vi "LDA_U16_data_header.vi"() -> (0 "Output string":string)   [LabVIEW 2018]
uses:
  Globals/Meas_global.vi
  Globals/LDA_meas_global_1.vi
  Globals/LDA_meas_global_2.vi
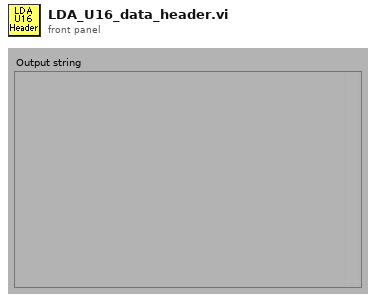
[diagram p1: front panel]
types:
  T1 = typedef "LDA_Setup.ctl" = cluster{"dimensions":enum16{"1D", "2D"}, "Sampling Rate Hz":dbl}
  T2 = typedef "BSA_Type.ctl" = enum16{"57N11", "BSA F60"}
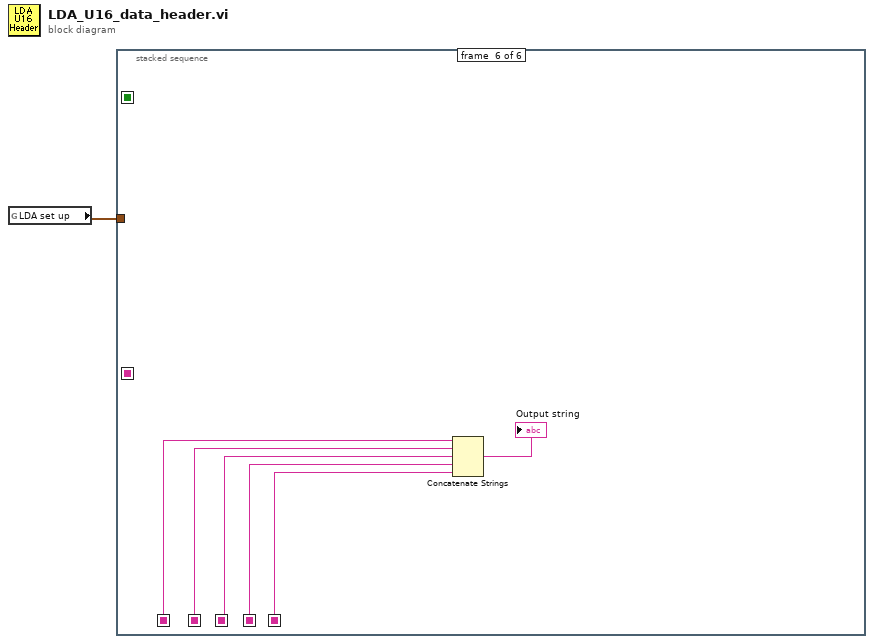
[diagram p0: block diagram]
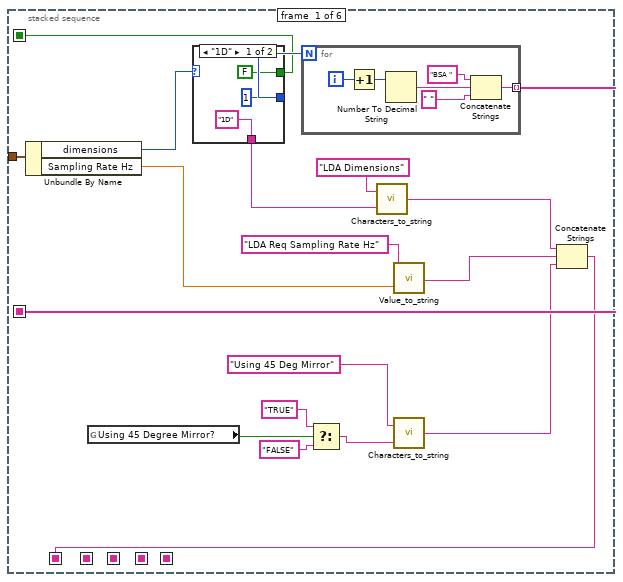
[diagram p2: hidden frame]
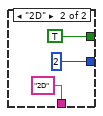
[diagram p3: hidden frame]
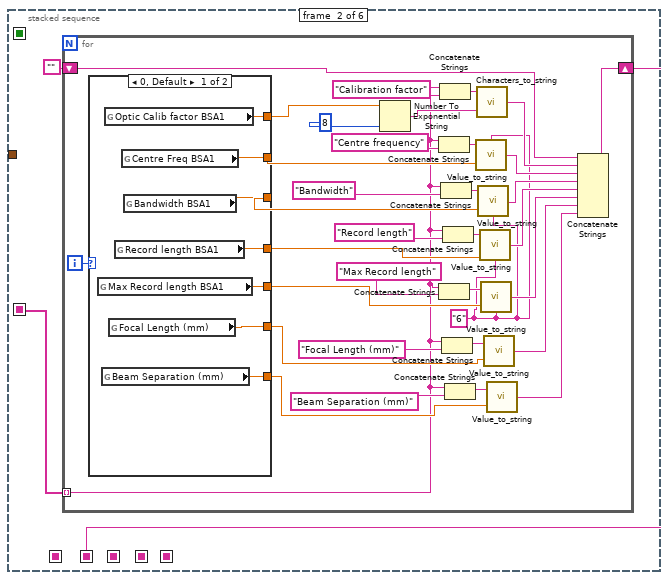
[diagram p4: hidden frame]
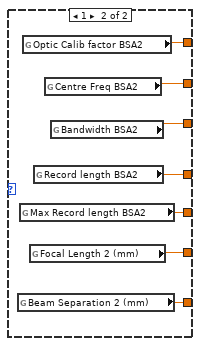
[diagram p5: hidden frame]
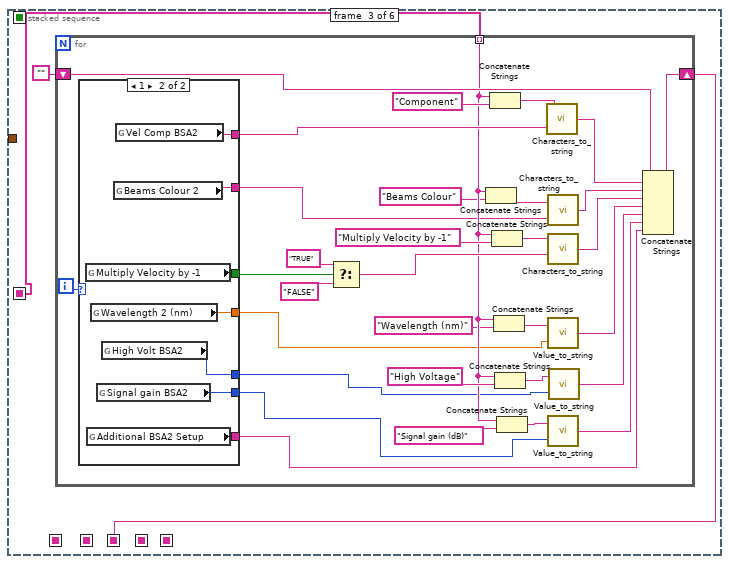
[diagram p6: hidden frame]
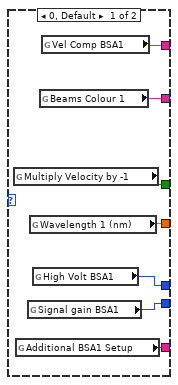
[diagram p7: hidden frame]
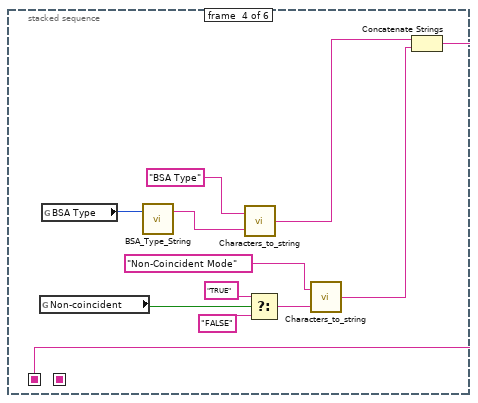
[diagram p8: hidden frame]
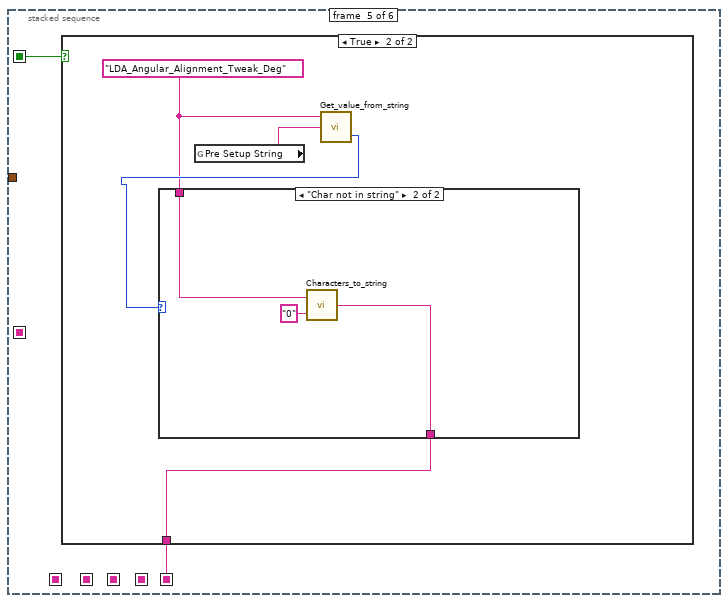
[diagram p9: hidden frame]
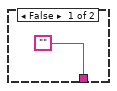
[diagram p10: hidden frame]
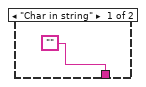
[diagram p11: hidden frame]
diagram:
  n1 = global read "Meas_global.vi" "LDA set up"() -> (w1:T1)
  n2 = stacked-sequence {
    seq-local: [_ w33 _ _ _ _] -> [_ _ _ _ _ w160]
    seq-local: [_ _ w85 _ _ _] -> [_ _ _ _ _ w159]
    seq-local: [w19 _ _ _ _ _] -> [_ w32 w84 _ _ _]
    seq-local: [_ _ _ w143 _ _] -> [_ _ _ _ _ w157]
    seq-local: [w2 _ _ _ _ _] -> [_ _ _ _ _ w156]
    seq-local: [_ _ _ _ w144 _] -> [_ _ _ _ _ w155]
    seq-local: [w11 _ _ _ _ _] -> [_ _ _ _ w145 _]
    tunnel: w1 -> [w10 _ _ _ _ _]
    frame #0 {
      n3 = Unbundle By Name(w10) -> ("dimensions"=w17:enum16{"1D", "2D"}, "Sampling Rate Hz"=w6:dbl)
      n4 = global read "LDA_meas_global_1.vi" "Using 45 Degree Mirror?"() -> (w13:bool)
      n5 = case shown="\"1D\"" w17 {
        tunnel: [1 2] -> w18
        tunnel: [FALSE TRUE] -> w11
        tunnel: ["1D" "2D"] -> w8
        frame "1D" {
        }
        frame "2D" {
        }
      }
      n6 = for {
        N: w18 -> [_]
        tunnel: [w28] -> w19 mode=indexing
        i -> [w26]
        n7 = Increment(x=w26) -> (x+1=w29:i32)
        n8 = Number To Decimal String(number=w29) -> (decimal integer string=w31:string)  [unwired: 1 out]
        n9 = Concatenate Strings("BSA ", w31, " ") -> (w28:string)
      }
      n10 = Select(t="TRUE", s=w13, f="FALSE") -> (s? t:f=w14:string)
      n11 = call "Characters_to_string.vi"("Characters to write"=w8, "Label for characters"="LDA Dimensions") -> ("Output string"=w5:string)
      n12 = call "Value_to_string.vi"("Value"=w6, "Label for value"="LDA Req Sampling Rate Hz") -> ("Output string"=w4:string)  [unwired: 1 in]
      n13 = call "Characters_to_string.vi"("Characters to write"=w14, "Label for characters"="Using 45 Deg Mirror") -> ("Output string"=w3:string)
      n14 = Concatenate Strings(w5, w4, w3) -> (w2:string)
    }
    frame #1 {
      n15 = for {
        shift-right: [w67] -> w33
        shift-left: "" -> [w68]
        tunnel: w32 -> [w35] mode=indexing
        i -> [w69]
        w47 = "6" ("precision")
        n16 = case shown="0, Default" w69 {
          tunnel: [w76 w80] -> w45
          tunnel: [w75 w81] -> w60
          tunnel: [w74 w82] -> w61
          tunnel: [w73 w83] -> w62
          tunnel: [w72 w79] -> w49
          tunnel: [w71 w77] -> w38
          tunnel: [w70 w78] -> w37
          frame 0, Default {
            n17 = global read "LDA_meas_global_1.vi" "Max Record length BSA1"() -> (w72:dbl)
            n18 = global read "LDA_meas_global_1.vi" "Beam Separation (mm)"() -> (w70:dbl)
            n19 = global read "LDA_meas_global_1.vi" "Optic Calib factor BSA1"() -> (w76:dbl)
            n20 = global read "LDA_meas_global_1.vi" "Focal Length (mm)"() -> (w71:dbl)
            n21 = global read "LDA_meas_global_1.vi" "Record length BSA1"() -> (w73:dbl)
            n22 = global read "LDA_meas_global_1.vi" "Centre Freq BSA1"() -> (w75:dbl)
            n23 = global read "LDA_meas_global_1.vi" "Bandwidth BSA1"() -> (w74:dbl)
          }
          frame 1 {
            n24 = global read "LDA_meas_global_2.vi" "Beam Separation 2 (mm)"() -> (w78:dbl)
            n25 = global read "LDA_meas_global_2.vi" "Max Record length BSA2"() -> (w79:dbl)
            n26 = global read "LDA_meas_global_2.vi" "Optic Calib factor BSA2"() -> (w80:dbl)
            n27 = global read "LDA_meas_global_2.vi" "Focal Length 2 (mm)"() -> (w77:dbl)
            n28 = global read "LDA_meas_global_2.vi" "Record length BSA2"() -> (w83:dbl)
            n29 = global read "LDA_meas_global_2.vi" "Centre Freq BSA2"() -> (w81:dbl)
            n30 = global read "LDA_meas_global_2.vi" "Bandwidth BSA2"() -> (w82:dbl)
          }
        }
        n31 = Number To Exponential String(number=w45, precision (6)=i16 8) -> (E-format string=w44:string)  [unwired: 2 out]
        n32 = Concatenate Strings(w35, "Centre frequency") -> (w65:string)
        n33 = Concatenate Strings(w35, "Max Record length") -> (w50:string)
        n34 = Concatenate Strings(w35, "Calibration factor") -> (w66:string)
        n35 = Concatenate Strings(w35, "Bandwidth") -> (w64:string)
        n36 = Concatenate Strings(w35, "Focal Length (mm)" ("Label for characters")) -> (w43:string)
        n37 = Concatenate Strings(w35, "Record length") -> (w63:string)
        n38 = Concatenate Strings(w35, "Beam Separation (mm)" ("Label for characters")) -> (w42:string)
        n39 = call "Value_to_string.vi"("precision"=w47, "Value"=w60, "Label for value"=w65) -> ("Output string"=w58:string)
        n40 = call "Characters_to_string.vi"("Characters to write"=w44, "Label for characters"=w66) -> ("Output string"=w59:string)
        n41 = call "Value_to_string.vi"("precision"=w47, "Value"=w61, "Label for value"=w64) -> ("Output string"=w57:string)
        n42 = call "Value_to_string.vi"("precision"=w47, "Value"=w62, "Label for value"=w63) -> ("Output string"=w52:string)
        n43 = call "Value_to_string.vi"("precision"=w47, "Value"=w49, "Label for value"=w50) -> ("Output string"=w48:string)
        n44 = call "Value_to_string.vi"("Value"=w38, "Label for value"=w43) -> ("Output string"=w39:string)  [unwired: 1 in]
        n45 = call "Value_to_string.vi"("Value"=w37, "Label for value"=w42) -> ("Output string"=w36:string)  [unwired: 1 in]
        n46 = Concatenate Strings(w68, w59, w58, w57, w52, w48, w39, w36) -> (w67:string)
      }
    }
    frame #2 {
      n47 = for {
        shift-right: [w116] -> w85
        shift-left: "" -> [w117]
        tunnel: w84 -> [w97] mode=indexing
        i -> [w118]
        n48 = case shown="1" w118 {
          tunnel: [w125 w132] -> w87
          tunnel: [w124 w131] -> w112
          tunnel: [w123 w130] -> w109
          tunnel: [w121 w129] -> w91
          tunnel: [w122 w128] -> w90
          tunnel: [w120 w127] -> w89
          tunnel: [w119 w126] -> w88
          frame 0, Default {
            n49 = global read "LDA_meas_global_1.vi" "Multiply Velocity by -1"() -> (w123:bool)
            n50 = global read "LDA_meas_global_1.vi" "Additional BSA1 Setup"() -> (w120:string)
            n51 = global read "LDA_meas_global_1.vi" "Signal gain BSA1"() -> (w121:i16)
            n52 = global read "LDA_meas_global_1.vi" "Wavelength 1 (nm)"() -> (w119:dbl)
            n53 = global read "LDA_meas_global_1.vi" "High Volt BSA1"() -> (w122:i16)
            n54 = global read "LDA_meas_global_1.vi" "Beams Colour 1"() -> (w125:string)
            n55 = global read "LDA_meas_global_1.vi" "Vel Comp BSA1"() -> (w124:string)
          }
          frame 1 {
            n56 = global read "LDA_meas_global_2.vi" "Multiply Velocity by -1"() -> (w130:bool)
            n57 = global read "LDA_meas_global_2.vi" "Additional BSA2 Setup"() -> (w127:string)
            n58 = global read "LDA_meas_global_2.vi" "Wavelength 2 (nm)"() -> (w126:dbl)
            n59 = global read "LDA_meas_global_2.vi" "Signal gain BSA2"() -> (w129:i16)
            n60 = global read "LDA_meas_global_2.vi" "High Volt BSA2"() -> (w128:i16)
            n61 = global read "LDA_meas_global_2.vi" "Beams Colour 2"() -> (w132:string)
            n62 = global read "LDA_meas_global_2.vi" "Vel Comp BSA2"() -> (w131:string)
          }
        }
        n63 = Select(t="TRUE" ("y"), s=w109, f="FALSE" ("y")) -> (s? t:f=w106:string)
        n64 = Concatenate Strings(w97, "Beams Colour" ("string")) -> (w103:string)
        n65 = Concatenate Strings(w97, "Component") -> (w115:string)
        n66 = Concatenate Strings(w97, "Multiply Velocity by -1") -> (w110:string)
        n67 = Concatenate Strings(w97, "Wavelength (nm)") -> (w102:string)
        n68 = Concatenate Strings(w97, "High Voltage") -> (w101:string)
        n69 = Concatenate Strings(w97, "Signal gain (dB)") -> (w100:string)
        n70 = call "Characters_to_string.vi"("Characters to write"=w112, "Label for characters"=w115) -> ("Output string"=w114:string)
        n71 = call "Characters_to_string.vi"("Characters to write"=w87, "Label for characters"=w103) -> ("Output string"=w104:string)
        n72 = call "Characters_to_string.vi"("Characters to write"=w106, "Label for characters"=w110) -> ("Output string"=w105:string)
        n73 = call "Value_to_string.vi"("Value"=w88, "Label for value"=w102) -> ("Output string"=w94:string)  [unwired: 1 in]
        n74 = call "Value_to_string.vi"("Value"=w91, "Label for value"=w100) -> ("Output string"=w96:string)  [unwired: 1 in]
        n75 = call "Value_to_string.vi"("Value"=w90, "Label for value"=w101) -> ("Output string"=w95:string)  [unwired: 1 in]
        n76 = Concatenate Strings(w117, w114, w104, w105, w94, w95, w96, w89) -> (w116:string)
      }
    }
    frame #3 {
      n77 = global read "LDA_meas_global_1.vi" "Non-coincident"() -> (w136:bool)
      n78 = global read "LDA_meas_global_1.vi" "BSA Type"() -> (w142:T2)
      n79 = call "BSA_Type_String.vi"("BSA Type"=w142) -> ("BSA String Out"=w141:string)  [unwired: 1 in, 1 out]
      n80 = call "Characters_to_string.vi"("Characters to write"=w141, "Label for characters"="BSA Type") -> ("Output string"=w140:string)
      n81 = Select(t="TRUE" ("y"), s=w136, f="FALSE" ("y")) -> (s? t:f=w135:string)
      n82 = call "Characters_to_string.vi"("Characters to write"=w135, "Label for characters"="Non-Coincident Mode") -> ("Output string"=w134:string)
      n83 = Concatenate Strings(w140, w134) -> (w143:string)
    }
    frame #4 {
      n84 = case shown="True" w145 {
        tunnel: ["" w147] -> w144
        frame False {
        }
        frame True {
          w148 = "LDA_Angular_Alignment_Tweak_Deg"
          n85 = global read "Meas_global.vi" "Pre Setup String"() -> (w150:string)
          n86 = call "Get_value_from_string.vi"("Input string"=w150, "Variable name"=w148) -> ("Status"=w149:enum16{"Char in string", "Char not in string"})  [unwired: 1 in, 1 out]
          n87 = case shown="\"Char not in string\"" w149 {
            tunnel: w148 -> [_ w154]
            tunnel: ["" w152] -> w147
            frame "Char in string" {
            }
            frame "Char not in string" {
              n88 = call "Characters_to_string.vi"("Characters to write"="0", "Label for characters"=w154) -> ("Output string"=w152:string)
            }
          }
        }
      }
    }
    frame #5 {
      n89 = Concatenate Strings(w156, w160, w159, w157, w155) -> (→"Output string":string)
    }
  }
